vi "Binary to ASCII - General.vi"(0 "Binary File & Path":path, 3 "error in":errorcluster) -> (10 "error out":errorcluster)   [LabVIEW 2013]
uses:
  <vilib>/Utility/file.llb/Write To Spreadsheet File (DBL).vi
panel:
  out "Test File Path":path
  out "Waveform Graph":dbl[][](graph)
  out "size(s)":i32[](array[numeric])
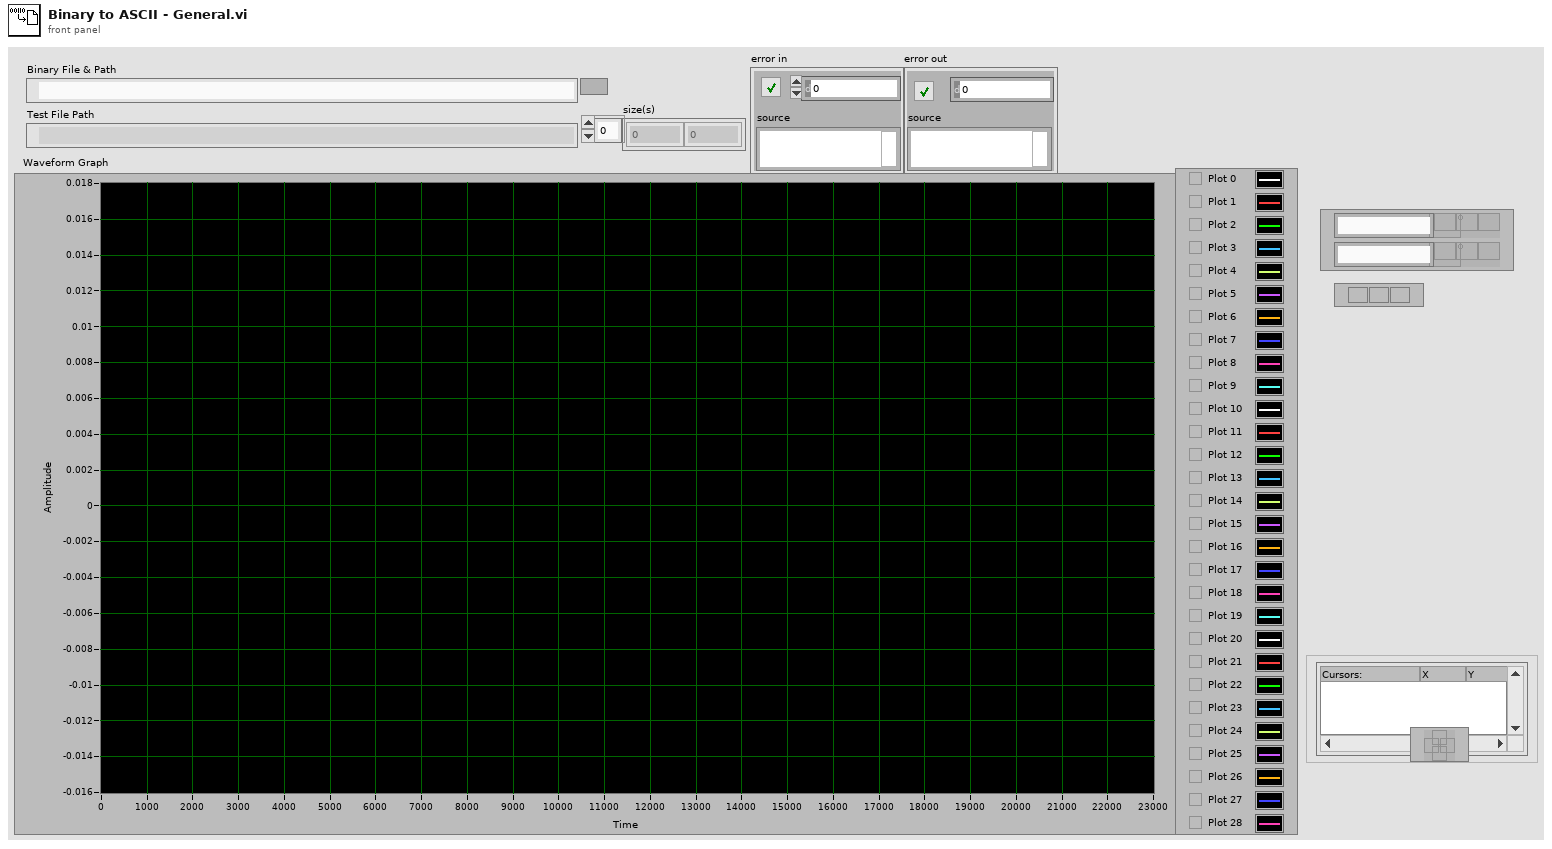
[diagram p1: front panel]
types:
  T1 = enum16{"open", "replace", "create", "open or create", "replace or create", "replace or create with confirmation"}
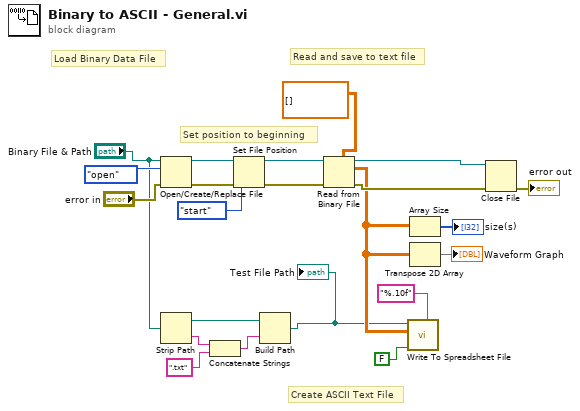
[diagram p0: block diagram]
diagram:
  # "Set position to beginning"
  # "Read and save to text file"
  # "Create ASCII Text File"
  # "Load Binary Data File"
  n1 = Open/Create/Replace File(file path (use dialog)="Binary File & Path", error in="error in", operation (0:open)=T1."open") -> (refnum out=w9:refnum<file>, error out=w11:errorcluster)  [unwired: 3 in, 1 out]
  n2 = Strip Path(path="Binary File & Path") -> (stripped path=w3:path, name=w5:string)
  n3 = Concatenate Strings(w5, ".txt" ("string")) -> (w2:string)
  n4 = Set File Position(refnum=w9, from (0:start)=enum16{"start", "end", "current"}."start", error in=w11) -> (refnum out=w8:refnum<file>, error out=w10:errorcluster)  [unwired: 1 in]
  n5 = Build Path(base path=w3, name or relative path=w2) -> (appended path=w1:path)
  "Test File Path" <- w1
  n6 = Read from Binary File(5:dbl[][] [], 8:w10, 11:w8) -> (0:w20:errorcluster, 2:w15:dbl[][], 3:w19:refnum<file>)  [unwired: 3 in, 1 out]
  n7 = call-poly <vilib>:"Write To Spreadsheet File.vi"("format (%.3f)"="%.10f", "append to file? (new file:F)"=FALSE, "2D data"=w15, "file path (dialog if empty)"=w1) -> ()  [unwired: 4 in, 1 out]
  n8 = Array Size(array=w15) -> (size(s)=→"size(s)":i32[])
  n9 = Transpose 2D Array(2D array=w15) -> (transposed array=→"Waveform Graph":dbl[][])
  n10 = Close File(refnum=w19, error in=w20) -> (error out=→"error out":errorcluster)  [unwired: 1 out]
